vi "Init External Sensors.vi"(8 "error in (no error)":errorcluster) -> (0 "error out":errorcluster)   [LabVIEW 2013]
uses:
  Names/Name Actions.ctl
  Transactions/Dataset Source.ctl
  Transactions/Dataset Type.ctl
  Apps/Yes No Button.ctl
  Transactions/Dataset Transaction Id.ctl
  Data Access Objects/Metadata/DAO Actions.ctl
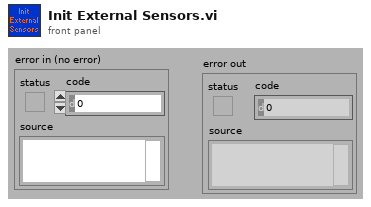
[diagram p1: front panel]
types:
  T1 = typedef "DAO Actions.ctl" = enum16{"Init", "Get", "Set"}
  T2 = typedef "Dataset Transaction Id.ctl" = cluster{"Dataset Source":T3, "Dataset Type":T4, "Hold":T5, "Volts":T5, "Tag":string}
  T3 = typedef "Dataset Source.ctl" = enum16{"Continuous", "Hold", "ED", "Volts", "Offsets", "Increments"}
  T4 = typedef "Dataset Type.ctl" = enum16{"LVDT", "Load Cell", "Actuator Command", "Servo Error", "Displacement Command", "Displacement", "Force"}
  T5 = typedef "Yes No Button.ctl" = bool
  T6 = typedef "Name Actions.ctl" = enum16{"Init", "Get Names", "Get Index"}
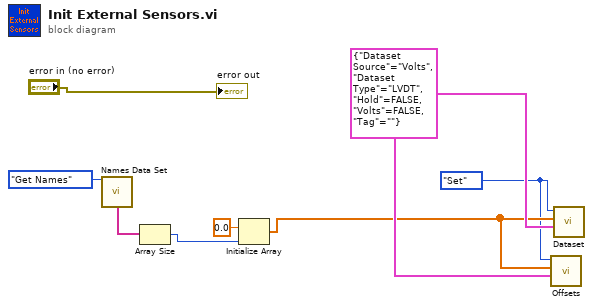
[diagram p0: block diagram]
diagram:
  w2 = DAO_Actions."Set" ("DAO Actions")
  w4 = T2 {"Dataset Source"=enum."Volts", "Dataset Type"=enum."LVDT", "Hold"=FALSE, "Volts"=FALSE, "Tag"=""} ("Dataset Trans Id")
  n1 = call "Names Data Set.vi"("Name Actions"=Name_Actions."Get Names") -> ("External Sensor Names"=w7:string[])  [unwired: 5 in, 9 out]
  n2 = Array Size(array=w7) -> (size(s)=w6:i32)
  n3 = Initialize Array(0.0, w6) -> (w3:dbl[])
  n4 = call "Offsets.vi"("Dataset Trans Id"=w4, "Data In"=w3, "DAO Actions"=w2) -> ()  [unwired: 6 in, 3 out]
  n5 = call "Dataset.vi"("Group ID"=w4, "Data In"=w3, "DAO Actions"=w2) -> ()  [unwired: 6 in, 3 out]
  "error out" <- "error in (no error)"
